vi "ratio_pixel2mil.vi"(10 "max corner in":dbl[][](array[numeric]), 11 "side length (mm)":dbl) -> (3 "ratio":dbl)   [LabVIEW 2017]
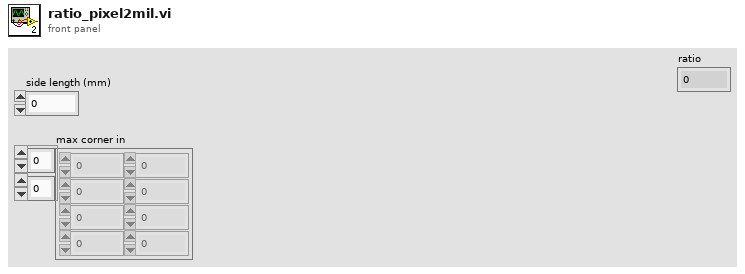
[diagram p1: front panel]
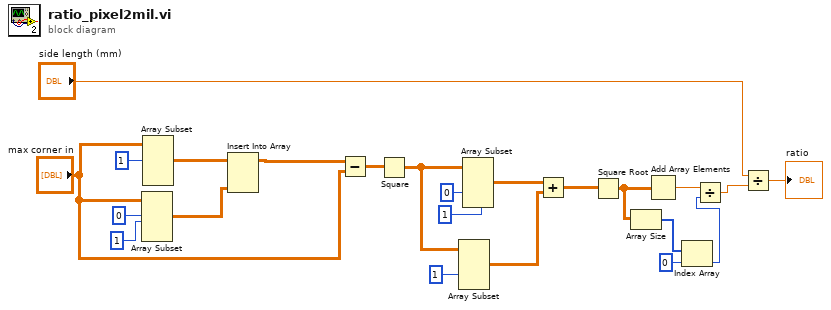
[diagram p0: block diagram]
diagram:
  n1 = Array Subset(array="max corner in", index (row)=0 ("length"), length (row)=1 ("length")) -> (w19:dbl[][])  [unwired: 2 in]
  n2 = Array Subset(array="max corner in", index (row)=1 ("index")) -> (w20:dbl[][])  [unwired: 3 in]
  n3 = Insert Into Array(array=w20, new element=w19) -> (w18:dbl[][])  [unwired: 2 in]
  n4 = Subtract(x=w18, y="max corner in") -> (x-y=w16:dbl[][])
  n5 = Square(x=w16) -> (x^2=w12:dbl[][])
  n6 = Array Subset(array=w12, index (col)=1 ("index")) -> (w10:dbl[][])  [unwired: 3 in]
  n7 = Array Subset(array=w12, index (col)=0 ("index"), length (col)=1 ("index")) -> (w11:dbl[][])  [unwired: 2 in]
  n8 = Add(x=w11, y=w10) -> (x+y=w9:dbl[][])
  n9 = Square Root(x=w9) -> (sqrt(x)=w7:dbl[][])
  n10 = Array Size(array=w7) -> (size(s)=w4:i32[])
  n11 = Add Array Elements(numeric array=w7) -> (sum=w8:dbl)
  n12 = Index Array(array=w4, index=0) -> (element=w2:i32)
  n13 = Divide(x=w8, y=w2) -> (x/y=w5:dbl)
  n14 = Divide(x="side length (mm)", y=w5) -> (x/y=→"ratio":dbl)
